vi "Empty All Notifier.vi"(8 "error in (no error)":errorcluster, 11 "Simple Map Notifier Controller in":refnum<class "Map Notifier Controller.lvclass">) -> (0 "error out":errorcluster, 3 "Simple Map Notifier Controller out":refnum<class "Map Notifier Controller.lvclass">)   [LabVIEW 2024, in "Map Notifier Controller.lvclass"]
uses:
  Map Notifier Controller.lvclass
  Map Notifier Controller.lvclass/Map Notifier Controller.ctl
  Ancestor Class/Actor Assistant/Notifier/Notifier.lvclass
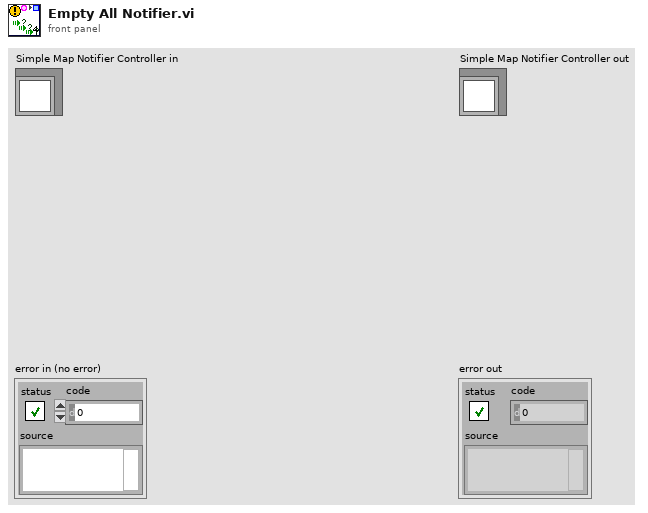
[diagram p1: front panel]
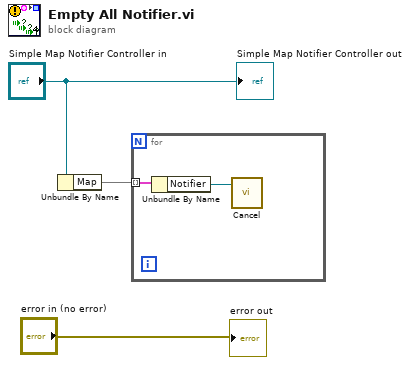
[diagram p0: block diagram]
diagram:
  n1 = Unbundle By Name("Simple Map Notifier Controller in") -> ("Map"=w2:map{i64, refnum<class "Notifier.lvclass">})
  n2 = for {
    tunnel: w2 -> [w5] mode=indexing
    n3 = Unbundle By Name(w5) -> ("Notifier"=w4:refnum<class "Notifier.lvclass">)
    n4 = call-dynamic "Cancel.vi"("Notifier in"=w4) -> ()  [unwired: 9 in, 2 out]
  }
  "error out" <- "error in (no error)"
  "Simple Map Notifier Controller out" <- "Simple Map Notifier Controller in"
